vi "Create Palette.vi"(9 "Palette Index":i32, 11 "Palette Lump":u8[](array[numeric])) -> (2 "Palette":u32[](array[colorbox]))   [LabVIEW 2017]
panel:
  # "https://doomwiki.org/wiki/PLAYPAL"
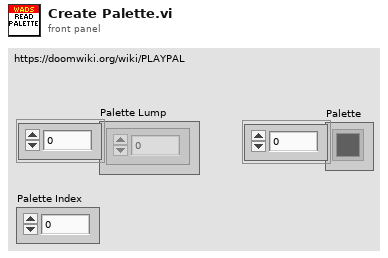
[diagram p1: front panel]
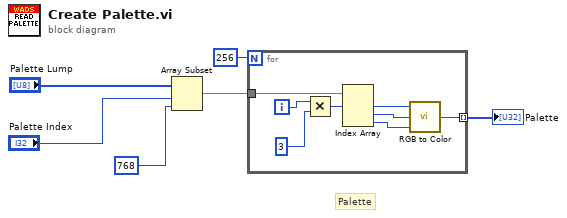
[diagram p0: block diagram]
diagram:
  # "Palette"
  n1 = Array Subset(array="Palette Lump", index="Palette Index", length=768 ("index")) -> (w4:u8[])
  n2 = for {
    N: 256 ("index") -> [_]
    tunnel: w4 -> [w14]
    tunnel: [w7] -> w1 mode=indexing
    i -> [w13]
    n3 = Multiply(x=w13, y=3 ("index")) -> (x*y=w12:i32)
    n4 = Index Array(array=w14, index #1=w12) -> (element #1=w10:u8, element #2=w9:u8, element #3=w8:u8)  [unwired: 2 in]
    n5 = call <vilib>:"RGB to Color.vi"("B"=w8, "G"=w9, "R"=w10) -> ("Color"=w7:u32)
  }
  "Palette" <- w1
